vi "Adv_Support_ParseXML.vi"(8 "error in (no error)":errorcluster, 10 "XML":string, 11 "SPE Refnum":refnum<file>) -> (0 "error out":errorcluster, 1 "ROI Info":T1, 2 "Frame Info":T2, 3 "SPE Refnum":refnum<file>)   [LabVIEW 2019, in "LightField Automation.lvclass"]
uses:
  LightField Automation.lvclass
  <vilib>/xml/Load XML String.vi
  <vilib>/xml/Close Reference(Node).vi
  <vilib>/xml/NI_XML.lvlib
  <resource>/objmgr/DOMUserDefRef.rc
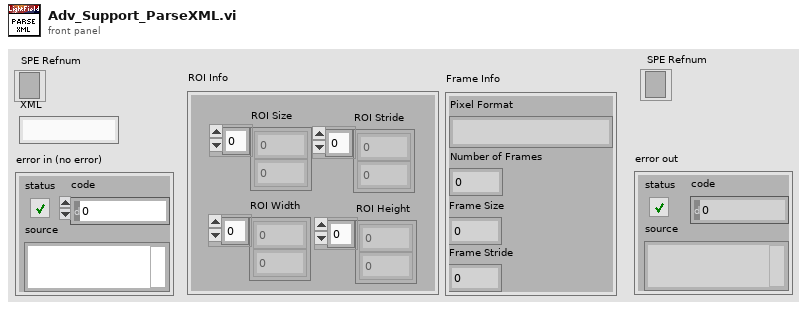
[diagram p1: front panel]
types:
  T1 = cluster{"ROI Height":i32[], "ROI Width":i32[], "ROI Stride":i32[], "ROI Size":i64[]}
  T2 = cluster{"Pixel Format":string, "Number of Frames":i32, "Frame Size":i32, "Frame Stride":i64}
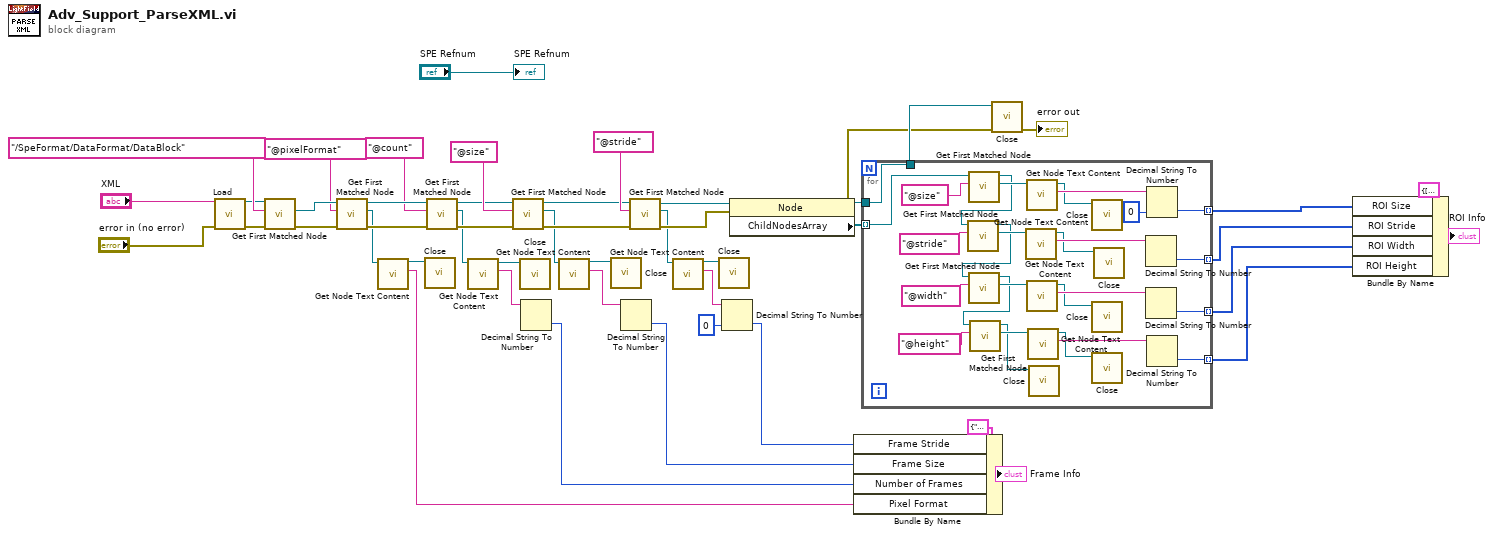
[diagram p0: block diagram]
diagram:
  n1 = call-poly <vilib>:"Load.vi"("XML string"="XML", "error in (no error)"="error in (no error)") -> ("DOM document out"=w18:refnum<k20>, "error out"=w21:errorcluster)  [unwired: 11 in, 1 out]
  n2 = call <vilib>:"Get First Matched Node.vi"("error in (no error)"=w21, "XPath expression"="/SpeFormat/DataFormat/DataBlock", "node in"=w18) -> ("error out"=w42:errorcluster, "node result"=w40:refnum<k20>)  [unwired: 6 in, 1 out]
  n3 = call <vilib>:"Get First Matched Node.vi"("error in (no error)"=w42, "XPath expression"="@pixelFormat", "node in"=w40) -> ("error out"=w45:errorcluster, "node result"=w41:refnum<k20>, "node out"=w43:refnum<k20>)  [unwired: 6 in]
  n4 = call <vilib>:"Get Node Text Content.vi"("node in"=w41) -> ("node text"=w12:string, "node out"=w20:refnum<k20>)  [unwired: 8 in, 1 out]
  n5 = call-poly <vilib>:"Close.vi"("node"=w20) -> ()  [unwired: 8 in, 1 out]
  n6 = call <vilib>:"Get First Matched Node.vi"("error in (no error)"=w45, "XPath expression"="@count", "node in"=w43) -> ("error out"=w33:errorcluster, "node result"=w24:refnum<k20>, "node out"=w31:refnum<k20>)  [unwired: 6 in]
  n7 = call <vilib>:"Get Node Text Content.vi"("node in"=w24) -> ("node text"=w25:string, "node out"=w23:refnum<k20>)  [unwired: 8 in, 1 out]
  n8 = call <vilib>:"Get First Matched Node.vi"("error in (no error)"=w33, "XPath expression"="@size", "node in"=w31) -> ("error out"=w34:errorcluster, "node result"=w27:refnum<k20>, "node out"=w32:refnum<k20>)  [unwired: 6 in]
  n9 = call-poly <vilib>:"Close.vi"("node"=w23) -> ()  [unwired: 8 in, 1 out]
  n10 = Decimal String To Number(string=w25) -> (number=w11:i32)  [unwired: 2 in, 1 out]
  n11 = call <vilib>:"Get Node Text Content.vi"("node in"=w27) -> ("node text"=w26:string, "node out"=w28:refnum<k20>)  [unwired: 8 in, 1 out]
  n12 = call-poly <vilib>:"Close.vi"("node"=w28) -> ()  [unwired: 8 in, 1 out]
  n13 = Decimal String To Number(string=w26) -> (number=w10:i32)  [unwired: 2 in, 1 out]
  n14 = call <vilib>:"Get First Matched Node.vi"("error in (no error)"=w34, "XPath expression"="@stride", "node in"=w32) -> ("error out"=w46:errorcluster, "node result"=w38:refnum<k20>, "node out"=w44:refnum<k20>)  [unwired: 6 in]
  n15 = call <vilib>:"Get Node Text Content.vi"("node in"=w38) -> ("node text"=w30:string, "node out"=w29:refnum<k20>)  [unwired: 8 in, 1 out]
  n16 = call-poly <vilib>:"Close.vi"("node"=w29) -> ()  [unwired: 8 in, 1 out]
  n17 = Decimal String To Number(string=w30, default (0L)=i64 0 ("default (0 I32)")) -> (number=w9:i64)  [unwired: 1 in, 1 out]
  n18 = property class="Node"(reference=w44, error in=w46) -> (reference out=w48:refnum<k20>, error out=w8:errorcluster, "ChildNodesArray"=w37:refnum<k20>[])
  n19 = Bundle By Name(cluster=T2 {"Pixel Format"="", "Number of Frames"=0, "Frame Size"=0, "Frame Stride"=0} ("Frame Info"), "Frame Stride"=w9, "Frame Size"=w10, "Number of Frames"=w11, "Pixel Format"=w12) -> (→"Frame Info":T2)
  n20 = for {
    tunnel: w37 -> [w68] mode=indexing
    tunnel: [w63] -> w1 mode=indexing
    tunnel: [w62] -> w2 mode=indexing
    tunnel: [w61] -> w3 mode=indexing
    tunnel: [w60] -> w4 mode=indexing
    tunnel: [w50] -> w49
    tunnel: w48 -> [w50]
    n21 = call <vilib>:"Get First Matched Node.vi"("XPath expression"="@size", "node in"=w68) -> ("node result"=w74:refnum<k20>, "node out"=w59:refnum<k20>)  [unwired: 7 in, 1 out]
    n22 = call <vilib>:"Get First Matched Node.vi"("XPath expression"="@stride", "node in"=w59) -> ("node result"=w75:refnum<k20>, "node out"=w58:refnum<k20>)  [unwired: 7 in, 1 out]
    n23 = call <vilib>:"Get First Matched Node.vi"("XPath expression"="@width", "node in"=w58) -> ("node result"=w72:refnum<k20>, "node out"=w57:refnum<k20>)  [unwired: 7 in, 1 out]
    n24 = call <vilib>:"Get First Matched Node.vi"("XPath expression"="@height", "node in"=w57) -> ("node result"=w69:refnum<k20>, "node out"=w56:refnum<k20>)  [unwired: 7 in, 1 out]
    n25 = call <vilib>:"Get Node Text Content.vi"("node in"=w75) -> ("node text"=w66:string, "node out"=w54:refnum<k20>)  [unwired: 8 in, 1 out]
    n26 = call <vilib>:"Get Node Text Content.vi"("node in"=w74) -> ("node text"=w67:string, "node out"=w55:refnum<k20>)  [unwired: 8 in, 1 out]
    n27 = call <vilib>:"Get Node Text Content.vi"("node in"=w72) -> ("node text"=w65:string, "node out"=w53:refnum<k20>)  [unwired: 8 in, 1 out]
    n28 = call <vilib>:"Get Node Text Content.vi"("node in"=w69) -> ("node text"=w64:string, "node out"=w52:refnum<k20>)  [unwired: 8 in, 1 out]
    n29 = call-poly <vilib>:"Close.vi"("node"=w56) -> ()  [unwired: 8 in, 1 out]
    n30 = call-poly <vilib>:"Close.vi"("node"=w55) -> ()  [unwired: 8 in, 1 out]
    n31 = call-poly <vilib>:"Close.vi"("node"=w53) -> ()  [unwired: 8 in, 1 out]
    n32 = call-poly <vilib>:"Close.vi"("node"=w52) -> ()  [unwired: 8 in, 1 out]
    n33 = call-poly <vilib>:"Close.vi"("node"=w54) -> ()  [unwired: 8 in, 1 out]
    n34 = Decimal String To Number(string=w66) -> (number=w61:i32)  [unwired: 2 in, 1 out]
    n35 = Decimal String To Number(string=w65) -> (number=w62:i32)  [unwired: 2 in, 1 out]
    n36 = Decimal String To Number(string=w67, default (0L)=i64 0 ("default (0 I32)")) -> (number=w60:i64)  [unwired: 1 in, 1 out]
    n37 = Decimal String To Number(string=w64) -> (number=w63:i32)  [unwired: 2 in, 1 out]
  }
  n38 = call-poly <vilib>:"Close.vi"("error in (no error)"=w8, "node"=w49) -> ("error out"=→"error out":errorcluster)  [unwired: 7 in]
  n39 = Bundle By Name(cluster=T1 {"ROI Height"=[], "ROI Width"=[], "ROI Stride"=[], "ROI Size"=[]} ("ROI Info"), "ROI Size"=w4, "ROI Stride"=w3, "ROI Width"=w2, "ROI Height"=w1) -> (→"ROI Info":T1)
  "SPE Refnum" <- "SPE Refnum"
